vi "LVIS_Measure.vi"(5 "LastEventMeas?":bool, 7 "LastTestMeas?":bool, 8 "Error In":errorcluster, 10 "Log Step?":bool, 11 "MeasInfo":T1) -> (0 "Error Out":errorcluster, 3 "Status":T2)   [LabVIEW 2015]
doc: "Determines the Measurement Info based on the LVIS_Settings file and passed in values, giving precedence to the file and deriving values where requested. Determine event, test and measurement status, verify all event data and sent to the Data Commander and Event Log if enabled."
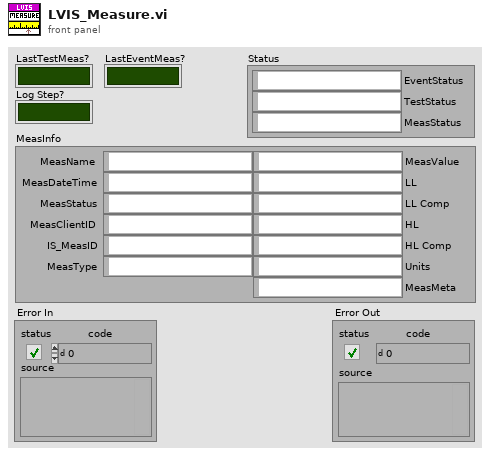
[diagram p1: front panel]
types:
  T1 = cluster{"MeasName":string, "MeasDateTime":string, "MeasStatus":string, "MeasClientID":string, "IS_MeasID":string, "MeasType":string, "MeasValue":string, "LL":string, "LL Comp":string, "HL":string, "HL Comp":string, "Units":string, "MeasMeta":string}
  T2 = cluster{"EventStatus":string, "TestStatus":string, "MeasStatus":string}
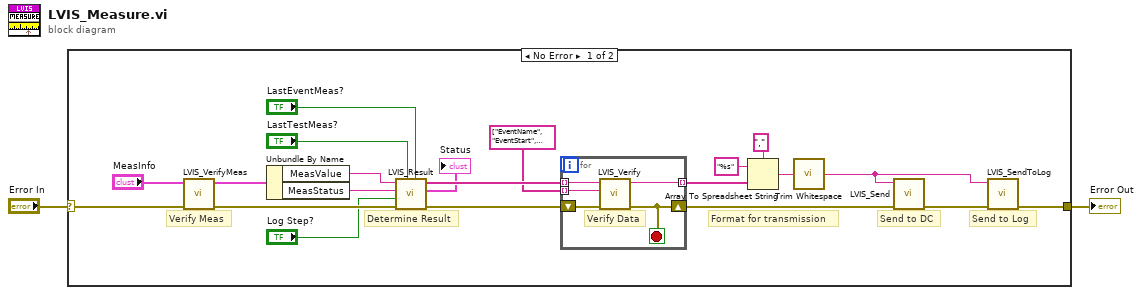
[diagram p0: block diagram]
diagram:
  n1 = case shown="No Error" "Error In" {
    selector: "Error In" -> [w23 w29]
    tunnel: [w8 w29] -> w1
    frame No Error {
      # "Send to Log"
      # "Verify Meas"
      # "Send to DC"
      # "Format for transmission"
      # "Determine Result"
      n2 = call "LVIS_VerifyMeas.vi"("Error In"=w23, "MeasInfoIn"="MeasInfo") -> ("Error Out"=w12:errorcluster, "MeasInfoOut"=w13:T1)  [unwired: 8 in]
      n3 = Unbundle By Name(w13) -> ("MeasValue"=w22:string, "MeasStatus"=w21:string)
      n4 = call "LVIS_Result.vi"("LastEventMeas?"="LastEventMeas?", "LastTestMeas?"="LastTestMeas?", "Error In"=w12, "Log Step?"="Log Step?", "Status"=w21, "Value"=w22) -> ("Error Out"=w11:errorcluster, "Result"=→"Status":T2, "IS_Data"=w18:string[])  [unwired: 3 in]
      n5 = for {
        tunnel: w18 -> [w27] mode=indexing
        tunnel: string[] ["EventName", "EventStart", "EventStop", "EventStatus", "EventClientID", "IS_EventID", "EventMeta", "ProductLine", "ProcessName", "Station", "Operator", "SN", "Model", "Manufacturer", "TestName", "TestDateTime", "TestStatus", "TestClientID", "IS_TestID", "TestMeta", "MeasName", "MeasDateTime", "MeasStatus", "MeasClientID", "IS_MeasID", "MeasType", "MeasValue", "LL", "LL Comp", "HL", "HL Comp", "Units", "MeasMeta"] ("appended array") -> [w26] mode=indexing
        shift-right: [w25] -> w10
        shift-left: w11 -> [w28]
        tunnel: [w24] -> w17 mode=indexing
        stop <- w25 stop-if-true
        # "Verify Data"
        n6 = call "LVIS_Verify.vi"("Error In"=w28, "Field Name"=w26, "Field Value In"=w27) -> ("Error Out"=w25:errorcluster, "Field Value Out"=w24:string)  [unwired: 7 in]
      }
      n7 = Array To Spreadsheet String(delimiter (Tab)=",", array=w17, 3:"%s" ("format string")) -> (spreadsheet string=w14:string)
      n8 = call <vilib>:"Trim Whitespace.vi"("string"=w14) -> ("trimmed string"=w7:string)  [unwired: 1 in]
      n9 = call "LVIS_Send.vi"("Error In"=w10, "Data In"=w7) -> ("Error Out"=w9:errorcluster)  [unwired: 9 in]
      n10 = call "LVIS_SendToLog.vi"("Error In"=w9, "EventData"=w7) -> ("Error Out"=w8:errorcluster)  [unwired: 9 in]
    }
    frame Error {
    }
  }
  "Error Out" <- w1
